vi "HeaderTable Columns Ratio.vi"(9 "Ratio right":sgl[](array[numeric]), 10 "Ratio left":sgl[](array[numeric]), 11 "Numerisch":i32) -> (2 "Array ratio":sgl[](array[numeric]), 3 "Array 1:1":sgl[](array[numeric]))   [LabVIEW 2020, in "PDF Interface.lvlib" / "PDF Interface Helper.lvlib"]
uses:
  PDF Interface Helper.lvlib
  Linearisierung V2/SpanEinstellungen/SpanEinstellungen.lvlib
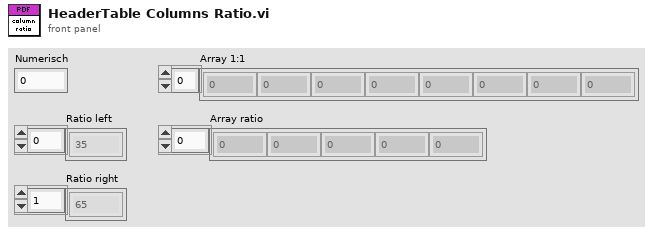
[diagram p1: front panel]
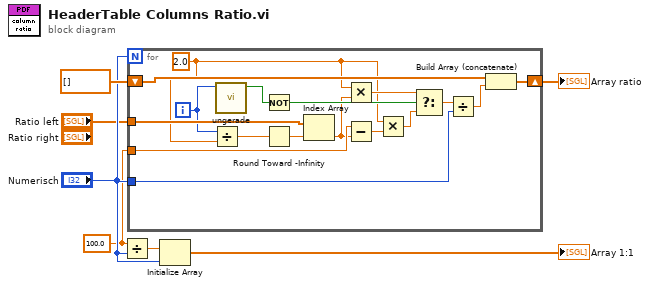
[diagram p0: block diagram]
diagram:
  w1 = sgl 100.0 ("Table Settings.Relative Column Widths (%)")
  n1 = Divide(x=w1, y="Numerisch") -> (x/y=w6:sgl)
  n2 = for {
    N: "Numerisch" -> [_]
    shift-right: [w21] -> w4
    shift-left: sgl[] [] ("x/y") -> [w20]
    tunnel: "Numerisch" -> [w22]
    tunnel: "Ratio left" -> [w15]
    tunnel: w1 -> [w16]
    i -> [w11]
    w9 = sgl 2.0 ("y")
    n3 = Divide(x=w11, y=w9) -> (x/y=w10:sgl)
    n4 = call "ungerade.vi"("Zahl"=w11) -> ("ungerade ?"=w24:bool)  [unwired: 10 in]
    n5 = Not(x=w24) -> (.not. x?=w18:bool)
    n6 = Round Toward -Infinity(1:w10) -> (0:w8:sgl)
    n7 = Index Array(array=w15, index=w8) -> (element=w12:sgl)
    n8 = Multiply(x=w9, y=w12) -> (x*y=w13:sgl)
    n9 = Subtract(x=w16, y=w12) -> (x-y=w17:sgl)
    n10 = Multiply(x=w9, y=w17) -> (x*y=w14:sgl)
    n11 = Select(t=w13, s=w18, f=w14) -> (s? t:f=w23:sgl)
    n12 = Divide(x=w23, y=w22) -> (x/y=w19:sgl)
    n13 = Build Array (concatenate)(w20, w19) -> (w21:sgl[])
  }
  "Array ratio" <- w4
  n14 = Initialize Array(w6, "Numerisch") -> (→"Array 1:1":sgl[])
